vi "CleanUp Control Logic.vi"(8 "error in (no error)":errorcluster, 10 "parameters":T1, 11 "Sequencer Module runtime in":refnum<class "Sequencer Module runtime.lvclass">) -> (0 "error out":errorcluster, 2 "Parameters allocation out":T1, 3 "Sequencer Module runtime out":refnum<class "Sequencer Module runtime.lvclass">)   [LabVIEW 2015, in "Sequencer Module runtime.lvclass"]
uses:
  Sequencer Module runtime.lvclass
  <vilib>/NI/Tag Bus/table/data table.ctl
  Sequencer Module runtime.lvclass/Sequencer Module runtime.ctl
  classes/Step/Execution/Step Status.ctl
  Sequencer State Enum.ctl
  classes/Step/Execution/Step.lvclass
  classes/Sequence/Execution/Sequence.lvclass
  <vilib>/NI/Tag Bus/table/data table.lvlib
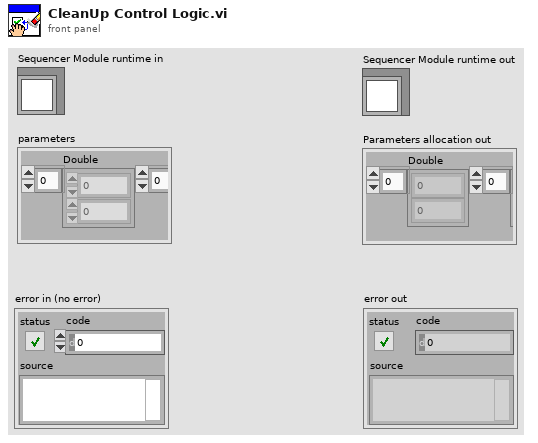
[diagram p1: front panel]
types:
  T1 = typedef "tag bus.lvlib/data table.lvlib/data table.ctl" = cluster{"Double":dbl[], "Single":sgl[], "I64":i64[], "I32":i32[], "I16":i16[], "I8":i8[], "U64":u64[], "U32":u32[], "U16":u16[], "U8":u8[], "Boolean":bool[], "String":string[], "Array of Double":cluster{"DBL Array":dbl[]}[], "Array of Single":cluster{"SGL Array":sgl[]}[], "Array of I64":cluster{"I64 Array":i64[]}[], "Array of I32":cluster{"I32 Array":i32[]}[], "Array of I16":cluster{"I16 Array":i16[]}[], "Array of I8":cluster{"I8 Array":i8[]}[], "Array of U64":cluster{"U64 Array":u64[]}[], "Array of U32":cluster{"U32 Array":u32[]}[], "Array of U16":cluster{"U16 Array":u16[]}[], "Array of U8":cluster{"U8 Array":u8[]}[], "Array of Boolean":cluster{"Boolean Array":bool[]}[], "Array of String":cluster{"String Array":string[]}[]}
  T2 = typedef "Sequencer Module runtime.lvclass/Sequencer Control.ctl" = cluster{"Start":bool, "Change Sequence":bool, "New Sequence":i32, "Pause":bool, "Abort":bool, "Terminate":bool}
  T3 = typedef "Sequencer Module runtime.lvclass/Sequencer Run Actions.ctl" = enum16{"Run", "Abort", "Pause", "Terminate"}
  T4 = typedef "Sequencer Module runtime.lvclass/Sequencer State Enum.ctl" = enum16{"Idle", "Paused", "Start Sequence", "Run Sequence", "CleanUp Sequence", "Generate Report"}
  T5 = typedef "Step.lvclass/Step Status.ctl" = enum16{"Start", "Passed", "Failed", "Error", "Done", "Terminated", "Skipped", "Running"}
  T6 = typedef "Step.lvclass/Step Flow Control.ctl" = enum16{"Next Step", "Jump"}
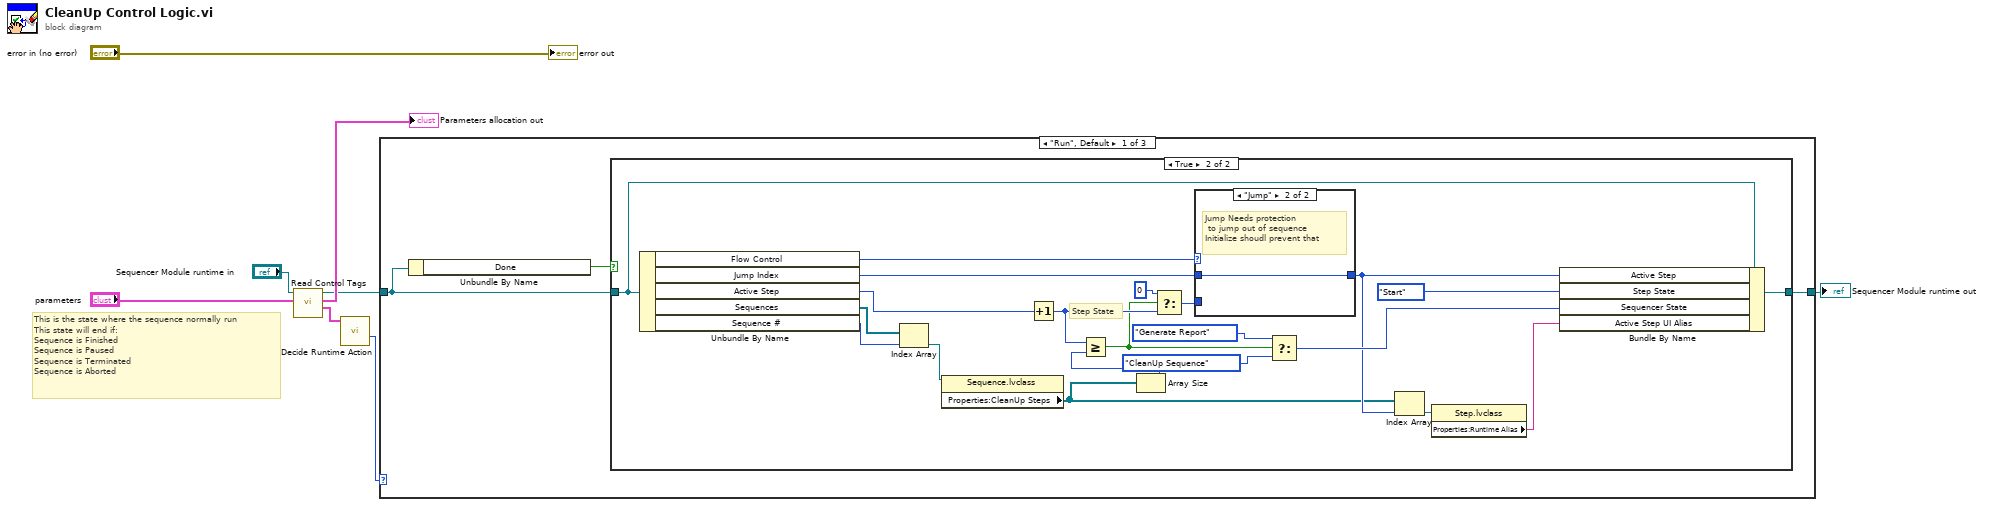
[diagram p0: block diagram]
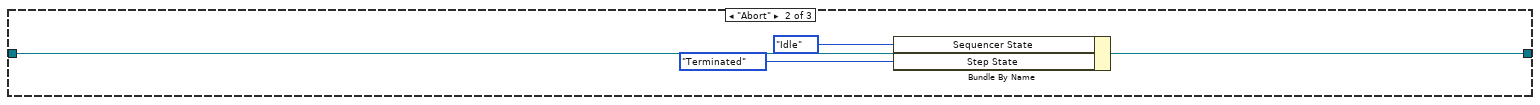
[diagram p4: hidden frame]
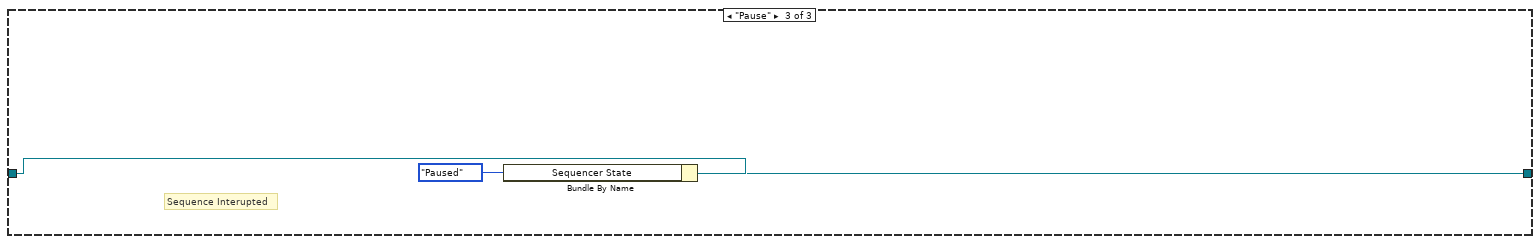
[diagram p5: hidden frame]
diagram:
  # "This is the state where the sequence normally run\nThis state will end if:\nSequence is Finished \nSequence is Paused\nSequence is Terminated \nSequence is Aborted"
  n1 = call "Read Control Tags.vi"("Paramaters  allocation in"="parameters", "Sequencer Module runtime in"="Sequencer Module runtime in") -> ("Sequence Control"=w5:T2, "Parameters allocation out"=→"Parameters allocation out":T1, "Sequencer Module runtime out"=w4:refnum<class "Sequencer Module runtime.lvclass">)  [unwired: 7 in]
  n2 = call "Decide Runtime Action.vi"("Sequence Control"=w5) -> ("Enum"=w2:T3)  [unwired: 10 in]
  n3 = case shown="\"Run\", Default" w2 {
    tunnel: w4 -> [w9 w39 w42]
    tunnel: [w10 w38 w41] -> w3
    frame "Run", Default {
      n4 = Unbundle By Name(w9) -> ("Done"=w11:bool)
      n5 = case shown="True" w11 {
        tunnel: w9 -> [w12 w29]
        tunnel: [w12 w33] -> w10
        frame False {
        }
        frame True {
          # "Step State"
          n6 = Unbundle By Name(w29) -> ("Flow Control"=w25:T6, "Jump Index"=w24:i32, "Active Step"=w28:i32, "Sequences"=w27:refnum<class "Sequence.lvclass">[], "Sequence #"=w26:i32)
          n7 = Index Array(array=w27, index=w26) -> (element=w15:refnum<class "Sequence.lvclass">)
          n8 = property class="Sequence.lvclass"(reference=w15) -> ("Properties:CleanUp Steps"=w14:refnum<class "Step.lvclass">[])  [unwired: 1 in, 2 out]
          n9 = Increment(x=w28) -> (x+1=w32:i32)
          n10 = Array Size(array=w14) -> (size(s)=w13:i32)
          n11 = Greater Or Equal?(x=w32, y=w13) -> (x >= y?=w22:bool)
          n12 = Select(t=0, s=w22, f=w32) -> (s? t:f=w30:i32)
          n13 = case shown="\"Jump\"" w25 {
            tunnel: w24 -> [_ w35]
            tunnel: w30 -> [w34 _]
            tunnel: [w34 w35] -> w18
            frame "Next Step", Default {
            }
            frame "Jump" {
              # "Jump Needs protection\n to jump out of sequence\nInitialize shoudl prevent that"
            }
          }
          n14 = Select(t=Sequencer_State_Enum."Generate Report" ("Sequencer State.Sequencer State"), s=w22, f=Sequencer_State_Enum."CleanUp Sequence") -> (s? t:f=w19:T4)
          n15 = Index Array(array=w14, index=w18) -> (element=w17:refnum<class "Step.lvclass">)
          n16 = property class="Step.lvclass"(reference=w17) -> ("Properties:Runtime Alias"=w16:string)  [unwired: 1 in, 2 out]
          n17 = Bundle By Name(cluster=w29, "Active Step"=w18, "Step State"=Step_Status."Start", "Sequencer State"=w19, "Active Step UI Alias"=w16) -> (w33:refnum<class "Sequencer Module runtime.lvclass">)
        }
      }
    }
    frame "Abort" {
      n18 = Bundle By Name(cluster=w39, "Sequencer State"=Sequencer_State_Enum."Idle" ("Sequencer State.Sequencer State"), "Step State"=Step_Status."Terminated" ("Sequencer State.Step State.Step State")) -> (w38:refnum<class "Sequencer Module runtime.lvclass">)
    }
    frame "Pause" {
      # "Sequence Interupted"
      n19 = Bundle By Name(cluster=w42, "Sequencer State"=Sequencer_State_Enum."Paused" ("Sequencer State.Sequencer State")) -> (w41:refnum<class "Sequencer Module runtime.lvclass">)
    }
  }
  "Sequencer Module runtime out" <- w3
  "error out" <- "error in (no error)"
